vi "Convert Controls to Cluster.vi"(9 "Control Array":string[][](array[string]), 11 "Controls Data":refnum<class "Control.lvclass">[](array[class])) -> (3 "Controls Data out":refnum<class "Control.lvclass">[](array[class]))   [LabVIEW 2020, in "VI Properties Editor.lvlib"]
doc: "Converts <B>Control Array</B> and <B>Indicator Array</B> to a cluster array to be used by back-end processes."
uses:
  VI Properties Editor.lvlib
  Classes/Control/Control.lvclass
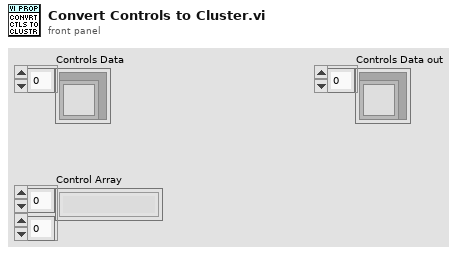
[diagram p1: front panel]
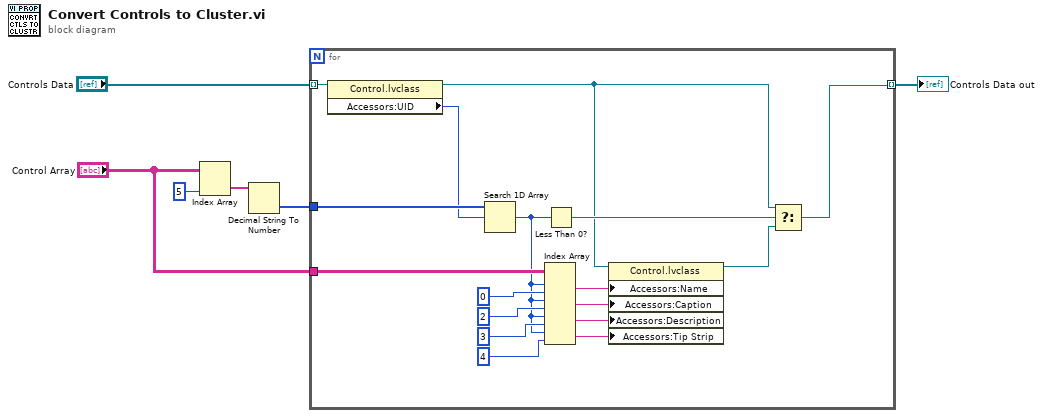
[diagram p0: block diagram]
diagram:
  n1 = Index Array(array="Control Array", index (col)=5 ("disabled index (col)")) -> (element=w3:string[])  [unwired: 1 in]
  n2 = Decimal String To Number(string=w3) -> (number=w2:i32[])  [unwired: 2 in, 1 out]
  n3 = for {
    tunnel: [w17] -> w6 mode=indexing
    tunnel: "Controls Data" -> [w9] mode=indexing
    tunnel: w2 -> [w23]
    tunnel: "Control Array" -> [w19]
    n4 = property class="Control.lvclass"(reference=w9) -> (reference out=w7:refnum<class "Control.lvclass">, "Accessors:UID"=w8:i32)  [unwired: 1 in, 1 out]
    n5 = Search 1D Array(1D array=w23, element=w8) -> (index of element=w15:i32)  [unwired: 1 in]
    n6 = Index Array(array=w19, index (row) #1=w15, index (col) #1=0 ("disabled index (col)"), index (row) #2=w15, index (col) #2=2 ("disabled index (col)"), index (row) #3=w15, index (col) #3=3 ("disabled index (col)"), index (row) #4=w15, index (col) #4=4 ("disabled index (col)")) -> (element #1=w13:string, element #2=w12:string, element #3=w11:string, element #4=w10:string)
    n7 = Less Than 0?(x=w15) -> (x < 0?=w18:bool)
    n8 = property class="Control.lvclass"(reference=w7, "Accessors:Name"=w13, "Accessors:Caption"=w12, "Accessors:Description"=w11, "Accessors:Tip Strip"=w10) -> (reference out=w14:refnum<class "Control.lvclass">)  [unwired: 1 in, 1 out]
    n9 = Select(t=w7, s=w18, f=w14) -> (s? t:f=w17:refnum<class "Control.lvclass">)
  }
  "Controls Data out" <- w6
